vi "Timer.vi"(7 "Reset":bool, 8 "error in (no error)":errorcluster) -> (0 "error out":errorcluster, 3 "Time (s)":dbl)   [LabVIEW 2016]
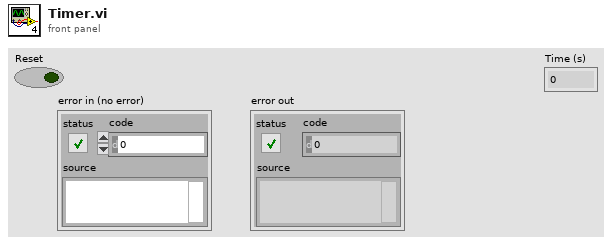
[diagram p1: front panel]
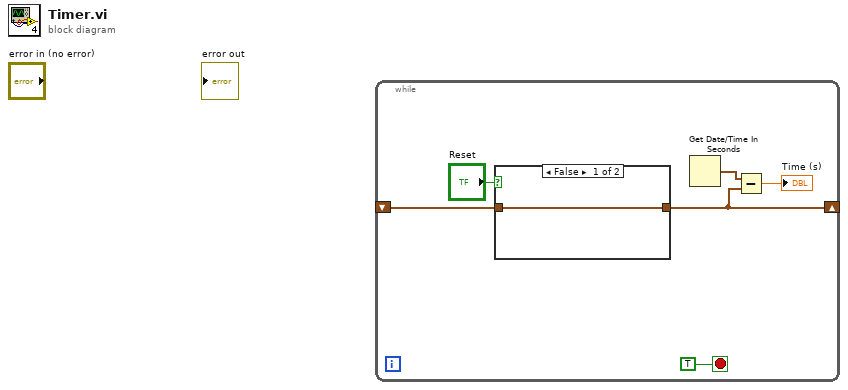
[diagram p0: block diagram]
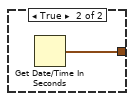
[diagram p2: hidden frame]
diagram:
  n1 = while {
    shift-right: [w2] -> _
    shift-left: _ -> [w4]
    stop <- TRUE stop-if-true
    n2 = case shown="False" "Reset" {
      tunnel: w4 -> [w7 _]
      tunnel: [w7 w8] -> w2
      frame False {
      }
      frame True {
        n3 = Get Date/Time In Seconds() -> (seconds since 1Jan1904=w8:timestamp)
      }
    }
    n4 = Get Date/Time In Seconds() -> (seconds since 1Jan1904=w3:timestamp)
    n5 = Subtract(x=w3, y=w2) -> (x-y=→"Time (s)":dbl)
  }
